vi "Close Sample Container Connections.vi"(8 "error in (no error)":errorcluster, 11 "Sample Line in":refnum<class "Sample Line.lvclass">) -> (0 "error out":errorcluster, 3 "Sample Line out":refnum<class "Sample Line.lvclass">)   [LabVIEW 2015, in "cRIO-Carbondioxide.lvlib" / "CO2-Actor.lvlib" / "Sample Line.lvclass"]
uses:
  Sample Line.lvclass
  Sample Line.lvclass/Sample Line.ctl
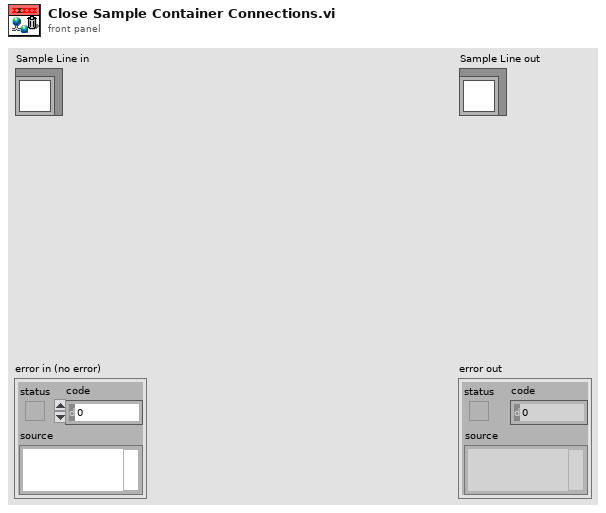
[diagram p1: front panel]
types:
  T1 = typedef "Sample Container.ctl" = cluster{"Sample In":refnum<k21>, "Sample Name":refnum<k21>, "Ti Cathode":refnum<k21>, "SampleQ":refnum<queue>}
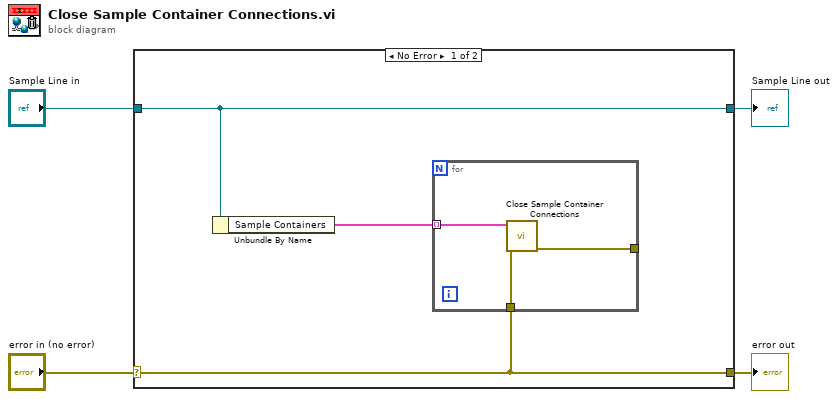
[diagram p0: block diagram]
diagram:
  n1 = case shown="No Error" "error in (no error)" {
    selector: "error in (no error)" -> [w6 w12]
    tunnel: [w6 w12] -> w3
    tunnel: [w7 w11] -> w1
    tunnel: "Sample Line in" -> [w7 w11]
    frame No Error {
      n2 = Unbundle By Name(w7) -> ("Sample Containers"=w5:T1[])
      n3 = for {
        tunnel: w5 -> [w10] mode=indexing
        tunnel: w6 -> [w9]
        tunnel: [w8] -> _
        n4 = call "Close Sample Container Connections.vi"("error in (no error)"=w9, "Container in"=w10) -> ("error out"=w8:errorcluster)  [unwired: 8 in, 1 out]
      }
    }
    frame Error {
    }
  }
  "error out" <- w3
  "Sample Line out" <- w1
